vi "Get isConnected.vi"(8 "error in (no error)":errorcluster, 11 "Instrument in":refnum<class "Instrument.lvclass">) -> (0 "error out":errorcluster, 2 "Instrument Address":bool, 3 "Instrument out":refnum<class "Instrument.lvclass">)   [LabVIEW 2017, in "Instrument.lvlib" / "Instrument.lvclass"]
doc: "Returns an Instruments Address as a string."
uses:
  Instrument.lvclass
  Instrument.lvclass/Instrument.ctl
  Properties/Instrument Properties.lvclass/Instrument Properties.ctl
  Properties/Instrument Properties.lvclass
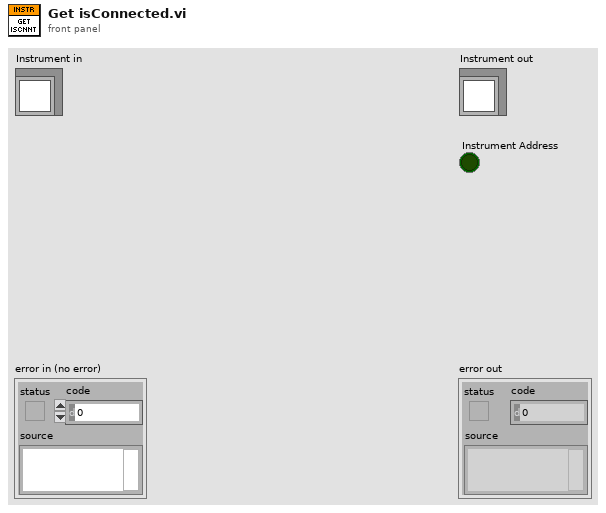
[diagram p1: front panel]
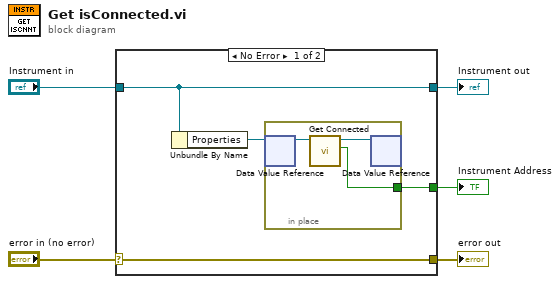
[diagram p0: block diagram]
diagram:
  n1 = case shown="No Error" "error in (no error)" {
    selector: "error in (no error)" -> [w9 w14]
    tunnel: [w9 w14] -> w4
    tunnel: [w8 w13] -> w2
    tunnel: "Instrument in" -> [w8 w13]
    tunnel: [w6 _] -> w1
    frame No Error {
      n2 = Unbundle By Name(w8) -> ("Properties"=w7:refnum<data-value>)
      n3 = in-place {
        in-place-border: [w12] -> w6
        n4 = in-place-dvr #1(w7) -> (w11:refnum<class "Instrument Properties.lvclass">)  [unwired: 1 out]
        n5 = call "Get Connected.vi"("Instrument Properties in"=w11) -> ("Connected"=w12:bool, "Instrument Properties out"=w10:refnum<class "Instrument Properties.lvclass">)  [unwired: 8 in, 1 out]
        n6 = in-place-dvr #1(w10) -> ()  [unwired: 2 out]
      }
    }
    frame Error {
    }
  }
  "error out" <- w4
  "Instrument out" <- w2
  "Instrument Address" <- w1
